vi "Main.vi"() -> ()   [LabVIEW 2014]
uses:
  Control 2.ctl
  <vilib>/MakerHub/LINX/Private/Type Defs/User Platform.ctl
  <vilib>/MakerHub/LINX/Private/Type Defs/Interface.ctl
  Geologico.ctl
  <vilib>/MakerHub/LINX/LMH-LINX.lvlib
panel:
  out "Sensado K":dbl
  out "Sensado P":dbl
  out "Sensado N":dbl
  in  "Stop Button":bool
  out "Sensado Ph":dbl
  in  "PIN PH":i8
  in  "Sensado PH":dbl
  in  "?":T1(tab)
  out "Nivel de humedad  2":string
  out "Porcentaje \nde humedad.":string
  out "Nivel de Humedad 2.":T2
  out "Miles de lumenes":dbl
  out "Temperatura":dbl
  out "Nivel de Humedad.":T2
  out "Estado":string
  out "Nivel de humedad":string
  out "Porcentaje de \nhumedad.":string
  in  "Serial Port":refnum<visa-resource-name>="N/A"
  in  "PIN Sensor °C":u8
  in  "Pin S. Humedad":u8
  in  "PIN \nFotoresistencia":u8
  in  "Arriba.":bool
  in  "Abajo":bool
  in  "Derecha":bool
  in  "Reversa":bool
  in  "Pause":bool
  in  "Velocidad":dbl(slide) scale=0.0..255.0
  in  "PIN Motores":T3
  in  "Ambiente":T4
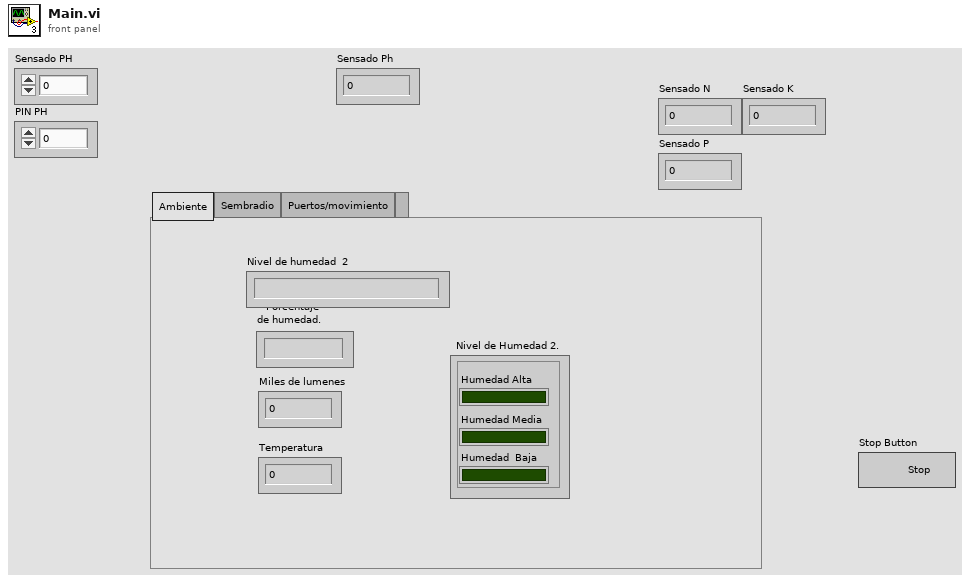
[diagram p1: front panel]
types:
  T1 = enum32{"Ambiente", "Sembradio", "Puertos/movimiento", ""}
  T2 = cluster{"Humedad Alta":bool, "Humedad  Baja":bool, "Humedad Media":bool}
  T3 = cluster{"PWM Channel":u8, "PWM Channel 2":u8, "PWM Channel 3":u8, "PWM Channel 4":u8}
  T4 = typedef "Control 2.ctl" = cluster{"Nivel de Humedad ":string, "Miles de lumenes":dbl, "Temperatura":dbl, "Estado":string, "Porcentaje de humedad":string}
  T5 = typedef "LMH-LINX.lvlib/Interface.ctl" = enum16{"Serial", "TCP"}
  T6 = typedef "LMH-LINX.lvlib/User Platform.ctl" = enum16{"Default", "LINX", "myRIO"}
  T7 = typedef "LMH-LINX.lvlib/LINX Ref.ctl" = cluster{"Platform":T8, "Interface":T5, "LINX Device Config":T9}
  T8 = typedef "LMH-LINX.lvlib/Platform.ctl" = enum16{"LINX", "myRIO"}
  T9 = typedef "LMH-LINX.lvlib/Device.lvlib/LINX Device Config.ctl" = cluster{"Interface":T5, "COM Port":refnum<visa-resource-name>, "TCP Configuration":T10, "Device Family":u8, "Device ID":u8, "Device Name":string, "TCP Ref":refnum<k5>, "Channels":T11}
  T10 = typedef "LMH-LINX.lvlib/Device.lvlib/TCP Config.ctl" = cluster{"IP Address":string, "Port":u16}
  T11 = typedef "LMH-LINX.lvlib/Channels.ctl" = cluster{"DI":u8[], "DO":u8[], "AI":u8[], "AO":u8[], "PWM":u8[], "QE":u8[], "UART":u8[], "I2C 2":u8[], "SPI":u8[], "CAN":u8[], "Servo":u8[], "AI Ref (V)":dbl, "AO Ref (V)":dbl, "AO Resolution (Bits)":u8}
  T12 = typedef "Geologico.ctl" = cluster{"String":string, "String 2":string, "Numeric Control":dbl}
  T13 = typedef "Semaphore RefNum" = refnum<k1>
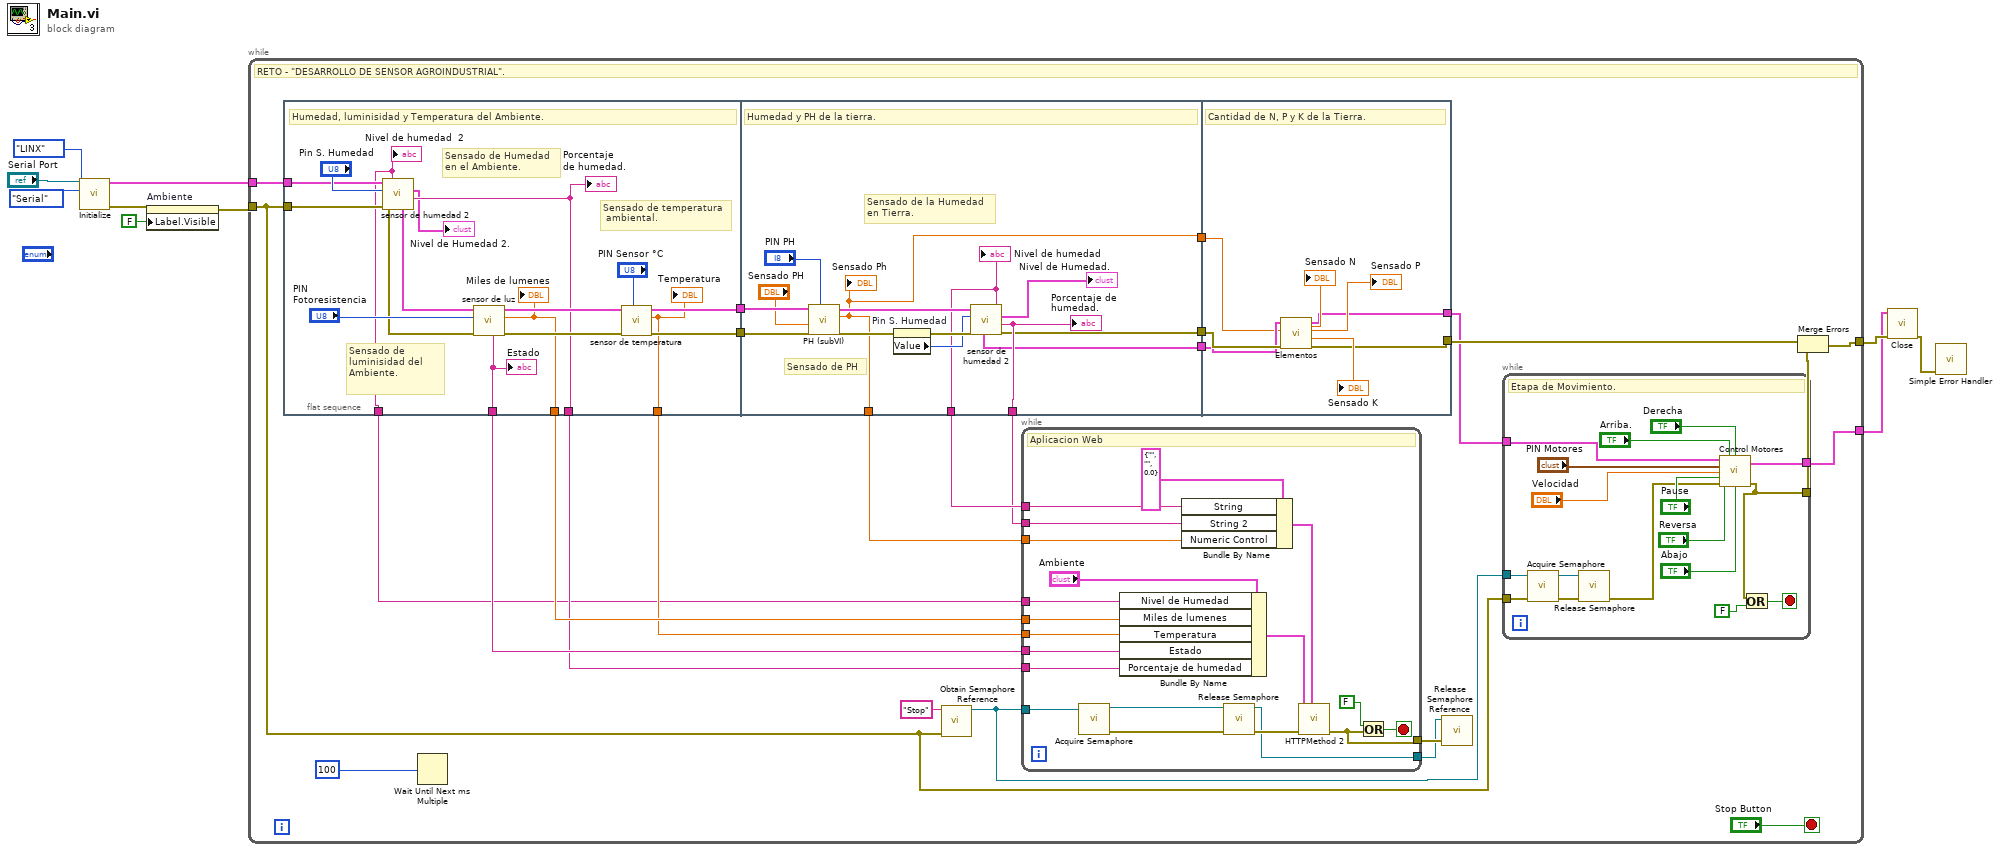
[diagram p0: block diagram]
diagram:
  n1 = call <vilib>:"Initialize.vi"("Serial Port"="Serial Port", "Interface"=Interface."Serial", "Platform"=User_Platform."LINX") -> ("Error Out"=w4:errorcluster, "LINX Ref"=w6:T7)  [unwired: 6 in, 1 out]
  n2 = property on="Ambiente" class="Clust (strict)"(error in=w4, "Label.Visible"=FALSE) -> (error out=w5:errorcluster)  [unwired: 1 in, 1 out]
  n3 = while {
    tunnel: w6 -> [w33]
    tunnel: w5 -> [w20]
    tunnel: [w13] -> w2
    tunnel: [w11] -> w1
    stop <- "Stop Button" stop-if-true
    # "RETO - \"DESARROLLO DE SENSOR AGROINDUSTRIAL\"."
    n4 = flat-sequence {
      tunnel: w33 -> [w89]
      tunnel: w20 -> [w88]
      tunnel: [w81] -> w35
      tunnel: [w80] -> w30
      tunnel: [w79] -> w34
      tunnel: [w78] -> w32
      tunnel: [w77] -> w31
      tunnel: [w76] -> w29
      tunnel: [w74] -> w28
      tunnel: w35 -> [w101]
      tunnel: w34 -> [w102]
      tunnel: [w91] -> w27
      tunnel: [w96] -> w25
      tunnel: [w94] -> w26
      tunnel: [w93] -> w24
      tunnel: [w92] -> w23
      tunnel: [w91] -> w16
      tunnel: w24 -> [w112]
      tunnel: w23 -> [w111]
      tunnel: w16 -> [w107]
      tunnel: [w106] -> w15
      tunnel: [w105] -> w12
      frame #0 {
        # "Sensado de temperatura\n ambiental."
        # "Sensado de \nluminisidad del \nAmbiente."
        # "Sensado de Humedad \nen el Ambiente."
        # "Humedad, luminisidad y Temperatura del Ambiente."
        n5 = call "sensor de humedad 2.vi"("Error In"=w88, "Pin S. Humedad"="Pin S. Humedad", "LINX Resource"=w89) -> ("Error Out"=w83:errorcluster, "Porcentaje de humedad"=w76:string, "Nivel de Humedad."=→"Nivel de Humedad 2.":T2, "LINX Resource 2"=w85:T7, "Nivel de humedad"=w74:string)  [unwired: 2 in]
        "Nivel de humedad  2" <- w74
        "Porcentaje \nde humedad." <- w76
        n6 = call "sensor de luz.vi"("Error In"=w83, "PIN Fotoresistencia"="PIN \nFotoresistencia", "LINX Resource"=w85) -> ("Error Out"=w82:errorcluster, "Miles de lumenes"=w78:dbl, "LINX Resource 2"=w84:T7, "Estado"=w80:string)  [unwired: 5 in]
        "Miles de lumenes" <- w78
        "Estado" <- w80
        n7 = call "sensor de temperatura.vi"("T sensor pin"="PIN Sensor °C", "Error In"=w82, "LINX Resource"=w84) -> ("Error Out"=w81:errorcluster, "Temperatura"=w77:dbl, "LINX Resource 2"=w79:T7)  [unwired: 6 in]
        "Temperatura" <- w77
      }
      frame #1 {
        # "Sensado de PH"
        # "Sensado de la Humedad \nen Tierra."
        # "Humedad y PH de la tierra."
        n8 = call "PH (subVI).vi"("PIN PH"="PIN PH", "Error In"=w101, "Sensado PH"="Sensado PH", "LINX Resource"=w102) -> ("Error Out"=w98:errorcluster, "Sensado Ph"=w91:dbl, "LINX Resource 2"=w97:T7)  [unwired: 5 in]
        "Sensado Ph" <- w91
        n9 = property on="Pin S. Humedad" class="DigNum (strict)"(error in=w98) -> (error out=w104:errorcluster, "Value"=w103:u8)  [unwired: 1 in, 1 out]
        n10 = call "sensor de humedad 2.vi"("Error In"=w104, "Pin S. Humedad"=w103, "LINX Resource"=w97) -> ("Error Out"=w93:errorcluster, "Porcentaje de humedad"=w96:string, "Nivel de Humedad."=→"Nivel de Humedad.":T2, "LINX Resource 2"=w92:T7, "Nivel de humedad"=w94:string)  [unwired: 2 in]
        "Nivel de humedad" <- w94
        "Porcentaje de \nhumedad." <- w96
      }
      frame #2 {
        # "Cantidad de N, P y K de la Tierra."
        n11 = call "Elementos.vi"("Error In"=w112, "Sensado PH"=w107, "LINX Resource"=w111) -> ("Error Out"=w106:errorcluster, "Sensado K"=→"Sensado K":dbl, "Sensado P"=→"Sensado P":dbl, "LINX Resource 2"=w105:T7, "Sensado N"=→"Sensado N":dbl)  [unwired: 4 in]
      }
    }
    n12 = Wait Until Next ms Multiple(millisecond multiple=u32 100) -> ()  [unwired: 1 out]
    n13 = call <vilib>:"Obtain Semaphore Reference.vi"("error in (no error)"=w20, "name (unnamed)"="Stop") -> ("semaphore"=w18:T13)  [unwired: 3 in, 2 out]
    n14 = while {
      tunnel: w32 -> [w54]
      tunnel: w31 -> [w53]
      tunnel: w30 -> [w52]
      tunnel: w29 -> [w51]
      tunnel: w28 -> [w49]
      tunnel: w27 -> [w46]
      tunnel: w26 -> [w48]
      tunnel: w25 -> [w47]
      tunnel: w18 -> [w43]
      tunnel: [w39] -> w21
      tunnel: [w38] -> w19
      stop <- w55 stop-if-true
      # "Aplicacion Web"
      n15 = call <vilib>:"Acquire Semaphore.vi"("semaphore"=w43) -> ("error out"=w41:errorcluster, "semaphore out"=w42:T13)  [unwired: 4 in, 1 out]
      n16 = Bundle By Name(cluster="Ambiente", "Nivel de Humedad"=w49, "Miles de lumenes"=w54, "Temperatura"=w53, "Estado"=w52, "Porcentaje de humedad"=w51) -> (w50:T4)
      n17 = Bundle By Name(cluster=T12 {"String"="", "String 2"="", "Numeric Control"=0.0} ("Control Geologico"), "String"=w48, "String 2"=w47, "Numeric Control"=w46) -> (w44:T12)
      n18 = call <vilib>:"Release Semaphore.vi"("error in (no error)"=w41, "semaphore"=w42) -> ("error out"=w40:errorcluster, "semaphore out"=w38:T13)  [unwired: 4 in]
      n19 = call "HTTPMethod 2.vi"("Control Geologico"=w44, "Error In"=w40, "Mediciones \nAmbietales"=w50) -> ("Error Out"=w39:errorcluster)  [unwired: 6 in, 2 out]
      n20 = Or(x=FALSE, y=w39) -> (x .or. y?=w55:bool)
    }
    n21 = call <vilib>:"Release Semaphore Reference.vi"("error in (no error)"=w21, "semaphore"=w19) -> ()  [unwired: 8 in, 2 out]
    n22 = while {
      tunnel: [w66] -> w11
      tunnel: w18 -> [w64]
      tunnel: w20 -> [w62]
      tunnel: [w58] -> w14
      tunnel: w12 -> [w57]
      stop <- w65 stop-if-true
      # "Etapa de Movimiento."
      n23 = call <vilib>:"Acquire Semaphore.vi"("error in (no error)"=w62, "semaphore"=w64) -> ("error out"=w61:errorcluster, "semaphore out"=w63:T13)  [unwired: 3 in, 1 out]
      n24 = call <vilib>:"Release Semaphore.vi"("error in (no error)"=w61, "semaphore"=w63) -> ("error out"=w60:errorcluster)  [unwired: 4 in, 1 out]
      n25 = call "Control Motores.vi"("LINX Resource"=w57, "Up Button"="Arriba.", "Next Button"="Derecha", "Cluster"="PIN Motores", "Velocidad"="Velocidad", "Pause Button"="Pause", "Error In"=w60, "Previous Button"="Reversa", "Down Button"="Abajo") -> ("LINX Resource 2"=w66:T7, "Error Out"=w58:errorcluster)  [unwired: 5 in]
      n26 = Or(x=w58, y=FALSE) -> (x .or. y?=w65:bool)
    }
    n27 = Merge Errors(w15, w14) -> (w13:errorcluster)
  }
  n28 = call <vilib>:"Close.vi"("Error In"=w2, "LINX Resource"=w1) -> ("Error Out"=w7:errorcluster)  [unwired: 8 in, 1 out]
  n29 = call <vilib>:"Simple Error Handler.vi"("error in (no error)"=w7) -> ()  [unwired: 4 in, 5 out]
